vi "etc_XCITE_SetXCStruct.vi"(8 "error in (no error)":errorcluster {"code" format="%x"}, 10 "XCiteStructure":T1, 11 "h":u64) -> (0 "error out":errorcluster {"code" format="%x"}, 2 "ErrorMessage":i32 format="%x", 3 "h out":u64)   [LabVIEW 2019, in "XCite.lvlib"]
doc: "Sends an Xcite structure to the device with various properties."
uses:
  XCite.lvlib
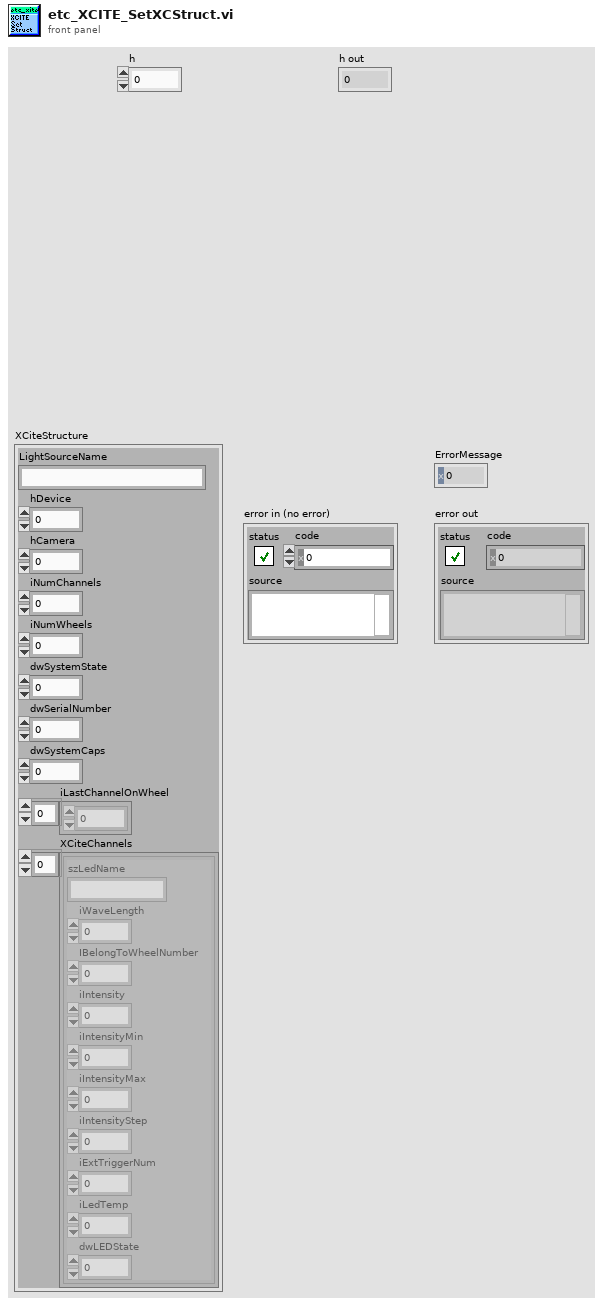
[diagram p1: front panel]
types:
  T1 = cluster{"LightSourceName":string, "hDevice":u64, "hCamera":u64, "iNumChannels":i32, "iNumWheels":i32, "dwSystemState":u32, "dwSerialNumber":u32, "dwSystemCaps":u32, "iLastChannelOnWheel":i32[], "XCiteChannels":cluster{"szLedName":string, "iWaveLength":i32, "IBelongToWheelNumber":i32, "iIntensity":i32, "iIntensityMin":i32, "iIntensityMax":i32, "iIntensityStep":i32, "iExtTriggerNum":i32, "iLedTemp":i32, "dwLEDState":u32}[]}
  T2 = cluster{"wSize":u16, "czLightSourceName":cluster{u8, u8, u8, u8, u8, u8, u8, u8, u8, u8, u8, u8, u8, u8, u8, u8, u8, u8, u8, u8, u8, u8, u8, u8, u8, u8, u8, u8, u8, u8}, "hDevice":u64, "hCamera":u64, "iNumChannels":i32, "iNumWheels":i32, "dwSystemState":u32, "dwSerialNumber":u32, "dwSystemCaps":u32, "iLastChannelOnWheel":cluster{i32, i32, i32, i32, i32}, "ZZdwDummy":cluster{u32, u32, u32, u32, u32, u32, u32, u32, u32, u32, u32, u32, u32, u32, u32, u32}, "XCiteChannels":cluster{"XCiteC_raw":cluster{"szLedName":cluster{u8, u8, u8, u8, u8, u8, u8, u8, u8, u8, u8, u8, u8, u8, u8, u8}, "iWaveLength":i32, "IBelongToWheelNumber":i32, "iIntensity":i32, "iIntensityMin":i32, "iIntensityMax":i32, "iIntensityStep":i32, "iExtTriggerNum":i32, "iLedTemp":i32, "dwLEDState":u32, "ZZdwdummy":cluster{u32, u32, u32, u32, u32, u32, u32, u32, u32, u32, u32, u32, u32, u32, u32, u32}}, "XCiteC_raw":cluster{"szLedName":cluster{u8, u8, u8, u8, u8, u8, u8, u8, u8, u8, u8, u8, u8, u8, u8, u8}, "iWaveLength":i32, "IBelongToWheelNumber":i32, "iIntensity":i32, "iIntensityMin":i32, "iIntensityMax":i32, "iIntensityStep":i32, "iExtTriggerNum":i32, "iLedTemp":i32, "dwLEDState":u32, "ZZdwdummy":cluster{u32, u32, u32, u32, u32, u32, u32, u32, u32, u32, u32, u32, u32, u32, u32, u32}}, "XCiteC_raw":cluster{"szLedName":cluster{u8, u8, u8, u8, u8, u8, u8, u8, u8, u8, u8, u8, u8, u8, u8, u8}, "iWaveLength":i32, "IBelongToWheelNumber":i32, "iIntensity":i32, "iIntensityMin":i32, "iIntensityMax":i32, "iIntensityStep":i32, "iExtTriggerNum":i32, "iLedTemp":i32, "dwLEDState":u32, "ZZdwdummy":cluster{u32, u32, u32, u32, u32, u32, u32, u32, u32, u32, u32, u32, u32, u32, u32, u32}}, "XCiteC_raw":cluster{"szLedName":cluster{u8, u8, u8, u8, u8, u8, u8, u8, u8, u8, u8, u8, u8, u8, u8, u8}, "iWaveLength":i32, "IBelongToWheelNumber":i32, "iIntensity":i32, "iIntensityMin":i32, "iIntensityMax":i32, "iIntensityStep":i32, "iExtTriggerNum":i32, "iLedTemp":i32, "dwLEDState":u32, "ZZdwdummy":cluster{u32, u32, u32, u32, u32, u32, u32, u32, u32, u32, u32, u32, u32, u32, u32, u32}}, "XCiteC_raw":cluster{"szLedName":cluster{u8, u8, u8, u8, u8, u8, u8, u8, u8, u8, u8, u8, u8, u8, u8, u8}, "iWaveLength":i32, "IBelongToWheelNumber":i32, "iIntensity":i32, "iIntensityMin":i32, "iIntensityMax":i32, "iIntensityStep":i32, "iExtTriggerNum":i32, "iLedTemp":i32, "dwLEDState":u32, "ZZdwdummy":cluster{u32, u32, u32, u32, u32, u32, u32, u32, u32, u32, u32, u32, u32, u32, u32, u32}}, "XCiteC_raw":cluster{"szLedName":cluster{u8, u8, u8, u8, u8, u8, u8, u8, u8, u8, u8, u8, u8, u8, u8, u8}, "iWaveLength":i32, "IBelongToWheelNumber":i32, "iIntensity":i32, "iIntensityMin":i32, "iIntensityMax":i32, "iIntensityStep":i32, "iExtTriggerNum":i32, "iLedTemp":i32, "dwLEDState":u32, "ZZdwdummy":cluster{u32, u32, u32, u32, u32, u32, u32, u32, u32, u32, u32, u32, u32, u32, u32, u32}}, "XCiteC_raw":cluster{"szLedName":cluster{u8, u8, u8, u8, u8, u8, u8, u8, u8, u8, u8, u8, u8, u8, u8, u8}, "iWaveLength":i32, "IBelongToWheelNumber":i32, "iIntensity":i32, "iIntensityMin":i32, "iIntensityMax":i32, "iIntensityStep":i32, "iExtTriggerNum":i32, "iLedTemp":i32, "dwLEDState":u32, "ZZdwdummy":cluster{u32, u32, u32, u32, u32, u32, u32, u32, u32, u32, u32, u32, u32, u32, u32, u32}}, "XCiteC_raw":cluster{"szLedName":cluster{u8, u8, u8, u8, u8, u8, u8, u8, u8, u8, u8, u8, u8, u8, u8, u8}, "iWaveLength":i32, "IBelongToWheelNumber":i32, "iIntensity":i32, "iIntensityMin":i32, "iIntensityMax":i32, "iIntensityStep":i32, "iExtTriggerNum":i32, "iLedTemp":i32, "dwLEDState":u32, "ZZdwdummy":cluster{u32, u32, u32, u32, u32, u32, u32, u32, u32, u32, u32, u32, u32, u32, u32, u32}}, "XCiteC_raw":cluster{"szLedName":cluster{u8, u8, u8, u8, u8, u8, u8, u8, u8, u8, u8, u8, u8, u8, u8, u8}, "iWaveLength":i32, "IBelongToWheelNumber":i32, "iIntensity":i32, "iIntensityMin":i32, "iIntensityMax":i32, "iIntensityStep":i32, "iExtTriggerNum":i32, "iLedTemp":i32, "dwLEDState":u32, "ZZdwdummy":cluster{u32, u32, u32, u32, u32, u32, u32, u32, u32, u32, u32, u32, u32, u32, u32, u32}}, "XCiteC_raw":cluster{"szLedName":cluster{u8, u8, u8, u8, u8, u8, u8, u8, u8, u8, u8, u8, u8, u8, u8, u8}, "iWaveLength":i32, "IBelongToWheelNumber":i32, "iIntensity":i32, "iIntensityMin":i32, "iIntensityMax":i32, "iIntensityStep":i32, "iExtTriggerNum":i32, "iLedTemp":i32, "dwLEDState":u32, "ZZdwdummy":cluster{u32, u32, u32, u32, u32, u32, u32, u32, u32, u32, u32, u32, u32, u32, u32, u32}}, "XCiteC_raw":cluster{"szLedName":cluster{u8, u8, u8, u8, u8, u8, u8, u8, u8, u8, u8, u8, u8, u8, u8, u8}, "iWaveLength":i32, "IBelongToWheelNumber":i32, "iIntensity":i32, "iIntensityMin":i32, "iIntensityMax":i32, "iIntensityStep":i32, "iExtTriggerNum":i32, "iLedTemp":i32, "dwLEDState":u32, "ZZdwdummy":cluster{u32, u32, u32, u32, u32, u32, u32, u32, u32, u32, u32, u32, u32, u32, u32, u32}}, "XCiteC_raw":cluster{"szLedName":cluster{u8, u8, u8, u8, u8, u8, u8, u8, u8, u8, u8, u8, u8, u8, u8, u8}, "iWaveLength":i32, "IBelongToWheelNumber":i32, "iIntensity":i32, "iIntensityMin":i32, "iIntensityMax":i32, "iIntensityStep":i32, "iExtTriggerNum":i32, "iLedTemp":i32, "dwLEDState":u32, "ZZdwdummy":cluster{u32, u32, u32, u32, u32, u32, u32, u32, u32, u32, u32, u32, u32, u32, u32, u32}}, "XCiteC_raw":cluster{"szLedName":cluster{u8, u8, u8, u8, u8, u8, u8, u8, u8, u8, u8, u8, u8, u8, u8, u8}, "iWaveLength":i32, "IBelongToWheelNumber":i32, "iIntensity":i32, "iIntensityMin":i32, "iIntensityMax":i32, "iIntensityStep":i32, "iExtTriggerNum":i32, "iLedTemp":i32, "dwLEDState":u32, "ZZdwdummy":cluster{u32, u32, u32, u32, u32, u32, u32, u32, u32, u32, u32, u32, u32, u32, u32, u32}}, "XCiteC_raw":cluster{"szLedName":cluster{u8, u8, u8, u8, u8, u8, u8, u8, u8, u8, u8, u8, u8, u8, u8, u8}, "iWaveLength":i32, "IBelongToWheelNumber":i32, "iIntensity":i32, "iIntensityMin":i32, "iIntensityMax":i32, "iIntensityStep":i32, "iExtTriggerNum":i32, "iLedTemp":i32, "dwLEDState":u32, "ZZdwdummy":cluster{u32, u32, u32, u32, u32, u32, u32, u32, u32, u32, u32, u32, u32, u32, u32, u32}}, "XCiteC_raw":cluster{"szLedName":cluster{u8, u8, u8, u8, u8, u8, u8, u8, u8, u8, u8, u8, u8, u8, u8, u8}, "iWaveLength":i32, "IBelongToWheelNumber":i32, "iIntensity":i32, "iIntensityMin":i32, "iIntensityMax":i32, "iIntensityStep":i32, "iExtTriggerNum":i32, "iLedTemp":i32, "dwLEDState":u32, "ZZdwdummy":cluster{u32, u32, u32, u32, u32, u32, u32, u32, u32, u32, u32, u32, u32, u32, u32, u32}}, "XCiteC_raw":cluster{"szLedName":cluster{u8, u8, u8, u8, u8, u8, u8, u8, u8, u8, u8, u8, u8, u8, u8, u8}, "iWaveLength":i32, "IBelongToWheelNumber":i32, "iIntensity":i32, "iIntensityMin":i32, "iIntensityMax":i32, "iIntensityStep":i32, "iExtTriggerNum":i32, "iLedTemp":i32, "dwLEDState":u32, "ZZdwdummy":cluster{u32, u32, u32, u32, u32, u32, u32, u32, u32, u32, u32, u32, u32, u32, u32, u32}}}}
  T3 = cluster{"szLedName":string, "iWaveLength":i32, "IBelongToWheelNumber":i32, "iIntensity":i32, "iIntensityMin":i32, "iIntensityMax":i32, "iIntensityStep":i32, "iExtTriggerNum":i32, "iLedTemp":i32, "dwLEDState":u32}[]
  T4 = cluster{"unsigned byte array[0]":u8, "unsigned byte array[1]":u8, "unsigned byte array[2]":u8, "unsigned byte array[3]":u8, "unsigned byte array[4]":u8, "unsigned byte array[5]":u8, "unsigned byte array[6]":u8, "unsigned byte array[7]":u8, "unsigned byte array[8]":u8, "unsigned byte array[9]":u8, "unsigned byte array[10]":u8, "unsigned byte array[11]":u8, "unsigned byte array[12]":u8, "unsigned byte array[13]":u8, "unsigned byte array[14]":u8, "unsigned byte array[15]":u8}
  T5 = cluster{"szLedName":cluster{u8, u8, u8, u8, u8, u8, u8, u8, u8, u8, u8, u8, u8, u8, u8, u8}, "iWaveLength":i32, "IBelongToWheelNumber":i32, "iIntensity":i32, "iIntensityMin":i32, "iIntensityMax":i32, "iIntensityStep":i32, "iExtTriggerNum":i32, "iLedTemp":i32, "dwLEDState":u32, "ZZdwdummy":cluster{u32, u32, u32, u32, u32, u32, u32, u32, u32, u32, u32, u32, u32, u32, u32, u32}}
  T6 = cluster{"unsigned byte array[0]":u8, "unsigned byte array[1]":u8, "unsigned byte array[2]":u8, "unsigned byte array[3]":u8, "unsigned byte array[4]":u8, "unsigned byte array[5]":u8, "unsigned byte array[6]":u8, "unsigned byte array[7]":u8, "unsigned byte array[8]":u8, "unsigned byte array[9]":u8, "unsigned byte array[10]":u8, "unsigned byte array[11]":u8, "unsigned byte array[12]":u8, "unsigned byte array[13]":u8, "unsigned byte array[14]":u8, "unsigned byte array[15]":u8, "unsigned byte array[16]":u8, "unsigned byte array[17]":u8, "unsigned byte array[18]":u8, "unsigned byte array[19]":u8, "unsigned byte array[20]":u8, "unsigned byte array[21]":u8, "unsigned byte array[22]":u8, "unsigned byte array[23]":u8, "unsigned byte array[24]":u8, "unsigned byte array[25]":u8, "unsigned byte array[26]":u8, "unsigned byte array[27]":u8, "unsigned byte array[28]":u8, "unsigned byte array[29]":u8}
  T7 = cluster{"[0]":cluster{"szLedName":cluster{u8, u8, u8, u8, u8, u8, u8, u8, u8, u8, u8, u8, u8, u8, u8, u8}, "iWaveLength":i32, "IBelongToWheelNumber":i32, "iIntensity":i32, "iIntensityMin":i32, "iIntensityMax":i32, "iIntensityStep":i32, "iExtTriggerNum":i32, "iLedTemp":i32, "dwLEDState":u32, "ZZdwdummy":cluster{u32, u32, u32, u32, u32, u32, u32, u32, u32, u32, u32, u32, u32, u32, u32, u32}}, "[1]":cluster{"szLedName":cluster{u8, u8, u8, u8, u8, u8, u8, u8, u8, u8, u8, u8, u8, u8, u8, u8}, "iWaveLength":i32, "IBelongToWheelNumber":i32, "iIntensity":i32, "iIntensityMin":i32, "iIntensityMax":i32, "iIntensityStep":i32, "iExtTriggerNum":i32, "iLedTemp":i32, "dwLEDState":u32, "ZZdwdummy":cluster{u32, u32, u32, u32, u32, u32, u32, u32, u32, u32, u32, u32, u32, u32, u32, u32}}, "[2]":cluster{"szLedName":cluster{u8, u8, u8, u8, u8, u8, u8, u8, u8, u8, u8, u8, u8, u8, u8, u8}, "iWaveLength":i32, "IBelongToWheelNumber":i32, "iIntensity":i32, "iIntensityMin":i32, "iIntensityMax":i32, "iIntensityStep":i32, "iExtTriggerNum":i32, "iLedTemp":i32, "dwLEDState":u32, "ZZdwdummy":cluster{u32, u32, u32, u32, u32, u32, u32, u32, u32, u32, u32, u32, u32, u32, u32, u32}}, "[3]":cluster{"szLedName":cluster{u8, u8, u8, u8, u8, u8, u8, u8, u8, u8, u8, u8, u8, u8, u8, u8}, "iWaveLength":i32, "IBelongToWheelNumber":i32, "iIntensity":i32, "iIntensityMin":i32, "iIntensityMax":i32, "iIntensityStep":i32, "iExtTriggerNum":i32, "iLedTemp":i32, "dwLEDState":u32, "ZZdwdummy":cluster{u32, u32, u32, u32, u32, u32, u32, u32, u32, u32, u32, u32, u32, u32, u32, u32}}, "[4]":cluster{"szLedName":cluster{u8, u8, u8, u8, u8, u8, u8, u8, u8, u8, u8, u8, u8, u8, u8, u8}, "iWaveLength":i32, "IBelongToWheelNumber":i32, "iIntensity":i32, "iIntensityMin":i32, "iIntensityMax":i32, "iIntensityStep":i32, "iExtTriggerNum":i32, "iLedTemp":i32, "dwLEDState":u32, "ZZdwdummy":cluster{u32, u32, u32, u32, u32, u32, u32, u32, u32, u32, u32, u32, u32, u32, u32, u32}}, "[5]":cluster{"szLedName":cluster{u8, u8, u8, u8, u8, u8, u8, u8, u8, u8, u8, u8, u8, u8, u8, u8}, "iWaveLength":i32, "IBelongToWheelNumber":i32, "iIntensity":i32, "iIntensityMin":i32, "iIntensityMax":i32, "iIntensityStep":i32, "iExtTriggerNum":i32, "iLedTemp":i32, "dwLEDState":u32, "ZZdwdummy":cluster{u32, u32, u32, u32, u32, u32, u32, u32, u32, u32, u32, u32, u32, u32, u32, u32}}, "[6]":cluster{"szLedName":cluster{u8, u8, u8, u8, u8, u8, u8, u8, u8, u8, u8, u8, u8, u8, u8, u8}, "iWaveLength":i32, "IBelongToWheelNumber":i32, "iIntensity":i32, "iIntensityMin":i32, "iIntensityMax":i32, "iIntensityStep":i32, "iExtTriggerNum":i32, "iLedTemp":i32, "dwLEDState":u32, "ZZdwdummy":cluster{u32, u32, u32, u32, u32, u32, u32, u32, u32, u32, u32, u32, u32, u32, u32, u32}}, "[7]":cluster{"szLedName":cluster{u8, u8, u8, u8, u8, u8, u8, u8, u8, u8, u8, u8, u8, u8, u8, u8}, "iWaveLength":i32, "IBelongToWheelNumber":i32, "iIntensity":i32, "iIntensityMin":i32, "iIntensityMax":i32, "iIntensityStep":i32, "iExtTriggerNum":i32, "iLedTemp":i32, "dwLEDState":u32, "ZZdwdummy":cluster{u32, u32, u32, u32, u32, u32, u32, u32, u32, u32, u32, u32, u32, u32, u32, u32}}, "[8]":cluster{"szLedName":cluster{u8, u8, u8, u8, u8, u8, u8, u8, u8, u8, u8, u8, u8, u8, u8, u8}, "iWaveLength":i32, "IBelongToWheelNumber":i32, "iIntensity":i32, "iIntensityMin":i32, "iIntensityMax":i32, "iIntensityStep":i32, "iExtTriggerNum":i32, "iLedTemp":i32, "dwLEDState":u32, "ZZdwdummy":cluster{u32, u32, u32, u32, u32, u32, u32, u32, u32, u32, u32, u32, u32, u32, u32, u32}}, "[9]":cluster{"szLedName":cluster{u8, u8, u8, u8, u8, u8, u8, u8, u8, u8, u8, u8, u8, u8, u8, u8}, "iWaveLength":i32, "IBelongToWheelNumber":i32, "iIntensity":i32, "iIntensityMin":i32, "iIntensityMax":i32, "iIntensityStep":i32, "iExtTriggerNum":i32, "iLedTemp":i32, "dwLEDState":u32, "ZZdwdummy":cluster{u32, u32, u32, u32, u32, u32, u32, u32, u32, u32, u32, u32, u32, u32, u32, u32}}, "[10]":cluster{"szLedName":cluster{u8, u8, u8, u8, u8, u8, u8, u8, u8, u8, u8, u8, u8, u8, u8, u8}, "iWaveLength":i32, "IBelongToWheelNumber":i32, "iIntensity":i32, "iIntensityMin":i32, "iIntensityMax":i32, "iIntensityStep":i32, "iExtTriggerNum":i32, "iLedTemp":i32, "dwLEDState":u32, "ZZdwdummy":cluster{u32, u32, u32, u32, u32, u32, u32, u32, u32, u32, u32, u32, u32, u32, u32, u32}}, "[11]":cluster{"szLedName":cluster{u8, u8, u8, u8, u8, u8, u8, u8, u8, u8, u8, u8, u8, u8, u8, u8}, "iWaveLength":i32, "IBelongToWheelNumber":i32, "iIntensity":i32, "iIntensityMin":i32, "iIntensityMax":i32, "iIntensityStep":i32, "iExtTriggerNum":i32, "iLedTemp":i32, "dwLEDState":u32, "ZZdwdummy":cluster{u32, u32, u32, u32, u32, u32, u32, u32, u32, u32, u32, u32, u32, u32, u32, u32}}, "[12]":cluster{"szLedName":cluster{u8, u8, u8, u8, u8, u8, u8, u8, u8, u8, u8, u8, u8, u8, u8, u8}, "iWaveLength":i32, "IBelongToWheelNumber":i32, "iIntensity":i32, "iIntensityMin":i32, "iIntensityMax":i32, "iIntensityStep":i32, "iExtTriggerNum":i32, "iLedTemp":i32, "dwLEDState":u32, "ZZdwdummy":cluster{u32, u32, u32, u32, u32, u32, u32, u32, u32, u32, u32, u32, u32, u32, u32, u32}}, "[13]":cluster{"szLedName":cluster{u8, u8, u8, u8, u8, u8, u8, u8, u8, u8, u8, u8, u8, u8, u8, u8}, "iWaveLength":i32, "IBelongToWheelNumber":i32, "iIntensity":i32, "iIntensityMin":i32, "iIntensityMax":i32, "iIntensityStep":i32, "iExtTriggerNum":i32, "iLedTemp":i32, "dwLEDState":u32, "ZZdwdummy":cluster{u32, u32, u32, u32, u32, u32, u32, u32, u32, u32, u32, u32, u32, u32, u32, u32}}, "[14]":cluster{"szLedName":cluster{u8, u8, u8, u8, u8, u8, u8, u8, u8, u8, u8, u8, u8, u8, u8, u8}, "iWaveLength":i32, "IBelongToWheelNumber":i32, "iIntensity":i32, "iIntensityMin":i32, "iIntensityMax":i32, "iIntensityStep":i32, "iExtTriggerNum":i32, "iLedTemp":i32, "dwLEDState":u32, "ZZdwdummy":cluster{u32, u32, u32, u32, u32, u32, u32, u32, u32, u32, u32, u32, u32, u32, u32, u32}}, "[15]":cluster{"szLedName":cluster{u8, u8, u8, u8, u8, u8, u8, u8, u8, u8, u8, u8, u8, u8, u8, u8}, "iWaveLength":i32, "IBelongToWheelNumber":i32, "iIntensity":i32, "iIntensityMin":i32, "iIntensityMax":i32, "iIntensityStep":i32, "iExtTriggerNum":i32, "iLedTemp":i32, "dwLEDState":u32, "ZZdwdummy":cluster{u32, u32, u32, u32, u32, u32, u32, u32, u32, u32, u32, u32, u32, u32, u32, u32}}}
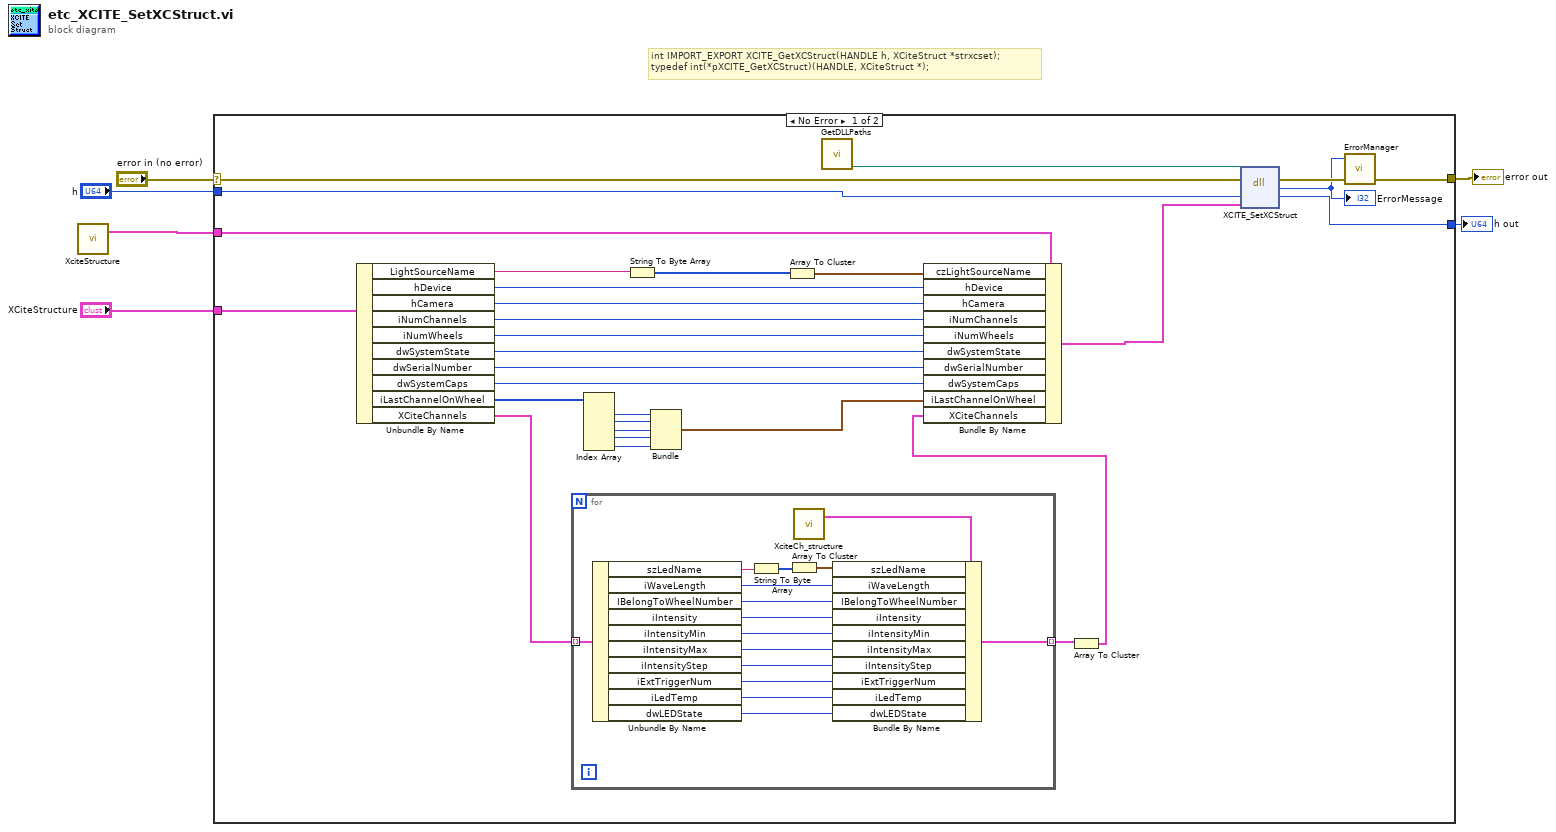
[diagram p0: block diagram]
diagram:
  # "int IMPORT_EXPORT XCITE_GetXCStruct(HANDLE h, XCiteStruct *strxcset);\ntypedef int(*pXCITE_GetXCStruct)(HANDLE, XCiteStruct *);"
  n1 = call "XciteStructure.vi"() -> ("XCiteStructure_raw"=w2:T2)  [unwired: 4 in, 3 out]
  n2 = case shown="No Error" "error in (no error)" {
    selector: "error in (no error)" -> [w36 w53]
    tunnel: [w34 w53] -> w6
    tunnel: "h" -> [w32 w52]
    tunnel: [w31 w52] -> w4
    tunnel: w2 -> [w21 _]
    tunnel: "XCiteStructure" -> [w22 _]
    frame No Error {
      n3 = Unbundle By Name(w22) -> ("LightSourceName"=w12:string, "hDevice"=w29:u64, "hCamera"=w28:u64, "iNumChannels"=w27:i32, "iNumWheels"=w26:i32, "dwSystemState"=w25:u32, "dwSerialNumber"=w24:u32, "dwSystemCaps"=w23:u32, "iLastChannelOnWheel"=w19:i32[], "XCiteChannels"=w20:T3)
      n4 = for {
        tunnel: w20 -> [w41] mode=indexing
        tunnel: [w42] -> w8 mode=indexing
        n5 = Unbundle By Name(w41) -> ("szLedName"=w40:string, "iWaveLength"=w51:i32, "IBelongToWheelNumber"=w50:i32, "iIntensity"=w49:i32, "iIntensityMin"=w48:i32, "iIntensityMax"=w47:i32, "iIntensityStep"=w46:i32, "iExtTriggerNum"=w45:i32, "iLedTemp"=w44:i32, "dwLEDState"=w43:u32)
        n6 = String To Byte Array(string=w40) -> (unsigned byte array=w39:u8[])
        n7 = Array To Cluster(array=w39) -> (cluster=w38:T4)
        n8 = call "XciteCh_structure.vi"() -> ("XCiteC_raw"=w37:T5)  [unwired: 4 in, 3 out]
        n9 = Bundle By Name(cluster=w37, "szLedName"=w38, "iWaveLength"=w51, "IBelongToWheelNumber"=w50, "iIntensity"=w49, "iIntensityMin"=w48, "iIntensityMax"=w47, "iIntensityStep"=w46, "iExtTriggerNum"=w45, "iLedTemp"=w44, "dwLEDState"=w43) -> (w42:T5)
      }
      n10 = Index Array(array=w19) -> (element #1=w14:i32, element #2=w15:i32, element #3=w16:i32, element #4=w17:i32, element #5=w18:i32)  [unwired: 5 in]
      n11 = String To Byte Array(string=w12) -> (unsigned byte array=w11:u8[])
      n12 = Bundle(w14, w15, w16, w17, w18) -> (w13:cluster{i32, i32, i32, i32, i32})  [unwired: 1 in]
      n13 = Array To Cluster(array=w11) -> (cluster=w10:T6)
      n14 = call "GetDLLPaths.vi"() -> ("etc_xcite_path"=w30:path)  [unwired: 8 in, 3 out]
      n15 = Array To Cluster(array=w8) -> (cluster=w7:T7)
      n16 = Bundle By Name(cluster=w21, "czLightSourceName"=w10, "hDevice"=w29, "hCamera"=w28, "iNumChannels"=w27, "iNumWheels"=w26, "dwSystemState"=w25, "dwSerialNumber"=w24, "dwSystemCaps"=w23, "iLastChannelOnWheel"=w13, "XCiteChannels"=w7) -> (w9:T2)
      n17 = dll-call lib="C:/LabVIEWDevFall2024/pco.labview/labview_sdk/runtime/bin64/etc_xcite.dll" fn="XCITE_SetXCStruct"(path in=w30, error in=w36, "h"=w32, "XciteStucture"=w9) -> (error out=w35:errorcluster, "return type"=w33:i32, "h"=w31:u64)  [unwired: 2 in, 1 out]
      "ErrorMessage" <- w33
      n18 = call "ErrorManager.vi"("error in (no error)"=w35, "error code"=w33) -> ("error out"=w34:errorcluster)  [unwired: 2 in, 1 out]
    }
    frame Error {
    }
  }
  "error out" <- w6
  "h out" <- w4
